vi "Read Multi Eval Meas EVM vs Chip Trace Results.vi"(7 "Result Type (Current)":i32(ring) items=["Current"=0, "Average"=1, "Maximum"=4], 8 "error in (no error)":errorcluster, 9 "Instance (1)":i32=1, 11 "VISA resource name":refnum<visa-resource-name>) -> (0 "error out":errorcluster, 1 "Reliability":i32, 2 "Results":dbl[](array[numeric]) format="%^.3e", 3 "VISA resource name out":refnum<visa-resource-name>)   [LabVIEW 2015, in "Rohde&Schwarz CMP LR WPAN Measurement.lvlib"]
doc: "Starts a single-shot measurement and returns the offset EVM vs chip traces. One value per two chips within the PSDU is returned.\n\nAttribute:\n-\n\nRemote-control commands:\nREAD:WPAN:MEAS<i>:MEValuation:TRACe:EVMChip[:OFFSet]:CURRent?\nREAD:WPAN:MEAS<i>:MEValuation:TRACe:EVMChip[:OFFSet]:AVERage?\nREAD:WPAN:MEAS<i>:MEValuation:TRACe:EVMChip[:OFFSet]:MAXimum?"
uses:
  <instrlib>/Rohde&Schwarz CMP LR WPAN Measurement/Rohde&Schwarz CMP LR WPAN Measurement.lvlib
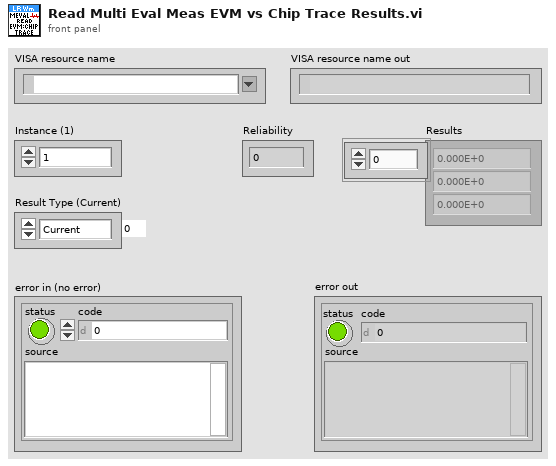
[diagram p1: front panel]
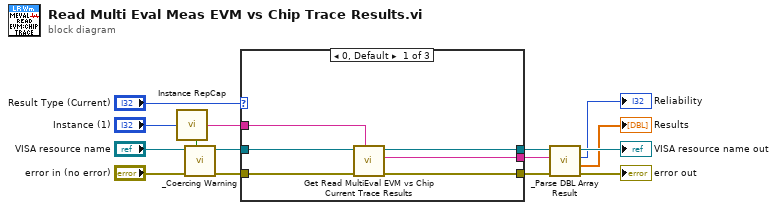
[diagram p0: block diagram]
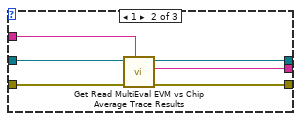
[diagram p2: hidden frame]
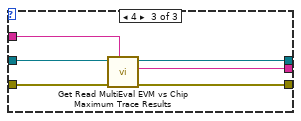
[diagram p3: hidden frame]
diagram:
  n1 = call <instrlib>:"Instance RepCap.vi"("Instance In"="Instance (1)") -> ("In Range?"=w14:bool, "RepCap Identifier Out"=w15:string)  [unwired: 1 in]
  n2 = call <instrlib>:"_Coercing Warning.vi"("In Range?"=w14, "error in (no error)"="error in (no error)", "VISA resource name"="VISA resource name") -> ("error out"=w11:errorcluster, "VISA resource name out"=w10:refnum<visa-resource-name>)  [unwired: 7 in]
  n3 = case shown="0, Default" "Result Type (Current)" {
    tunnel: w15 -> [w21 w27 w33]
    tunnel: w10 -> [w20 w26 w31]
    tunnel: w11 -> [w19 w25 w32]
    tunnel: [w16 w22 w28] -> w8
    tunnel: [w17 w23 w29] -> w5
    tunnel: [w18 w24 w30] -> w2
    frame 0, Default {
      n4 = call "Get Read MultiEval EVM vs Chip Current Trace Results"("Repeated Capabilities"=w21, "error in (no error)"=w19, "instrument handle"=w20) -> ("error out"=w17:errorcluster, "Read MultiEval EVM vs Chip Current Trace Results"=w18:string, "instrument handle out"=w16:refnum<visa-resource-name>)  [unwired: 6 in]
    }
    frame 1 {
      n5 = call "Get Read MultiEval EVM vs Chip Average Trace Results"("Repeated Capabilities"=w27, "error in (no error)"=w25, "instrument handle"=w26) -> ("error out"=w23:errorcluster, "Read MultiEval EVM vs Chip Average Trace Results"=w24:string, "instrument handle out"=w22:refnum<visa-resource-name>)  [unwired: 6 in]
    }
    frame 4 {
      n6 = call "Get Read MultiEval EVM vs Chip Maximum Trace Results"("Repeated Capabilities"=w33, "error in (no error)"=w32, "instrument handle"=w31) -> ("error out"=w29:errorcluster, "Read MultiEval EVM vs Chip Maximum Trace Results"=w30:string, "instrument handle out"=w28:refnum<visa-resource-name>)  [unwired: 6 in]
    }
  }
  n7 = call <instrlib>:"_Parse DBL Array Result.vi"("error in (no error)"=w5, "Input String"=w2, "VISA resource name"=w8) -> ("error out"=→"error out":errorcluster, "Results"=→"Results":dbl[], "Reliability"=→"Reliability":i32, "VISA resource name out"=→"VISA resource name out":refnum<visa-resource-name>)  [unwired: 5 in]
